vi "RTS Write Test Sequence.vi"(6 "Station Number":u16=1 min=1 max=8 step=1, 8 "Error In":errorcluster, 10 "Station Settings.Chamber Test Pattern":T1, 11 "Current Config File":T2 {"Chamber 1-1"."Start Time" format="%<%X\n%x>T"; "Chamber 1-1"."End Time" format="%<%X\n%x>T"; "Chamber 1-2"."Start Time" format="%<%X\n%x>T"; "Chamber 1-2"."End Time" format="%<%X\n%x>T"; "Chamber 1-3"."Start Time" format="%<%X\n%x>T"; "Chamber 1-3"."End Time" format="%<%X\n%x>T"}) -> (0 "Error Out":errorcluster)   [LabVIEW 2020]
uses:
  Type Definitions/RTS Door Op Data.ctl
  Type Definitions/RTS Door Ops Client.ctl
  Type Definitions/RTS Door Opening Schedule.ctl
  Type Definitions/RTS Door Ops Sequence.ctl
  Type Definitions/RTS Standard Door Opening Test.ctl
  Type Definitions/RTS Test Pattern.ctl
  <vilib>/Utility/config.llb/NI_LVConfig.lvlib
panel:
  # "Chamber Conditions:"
  # "Chamber Conditions:"
  # "Chamber Conditions:"
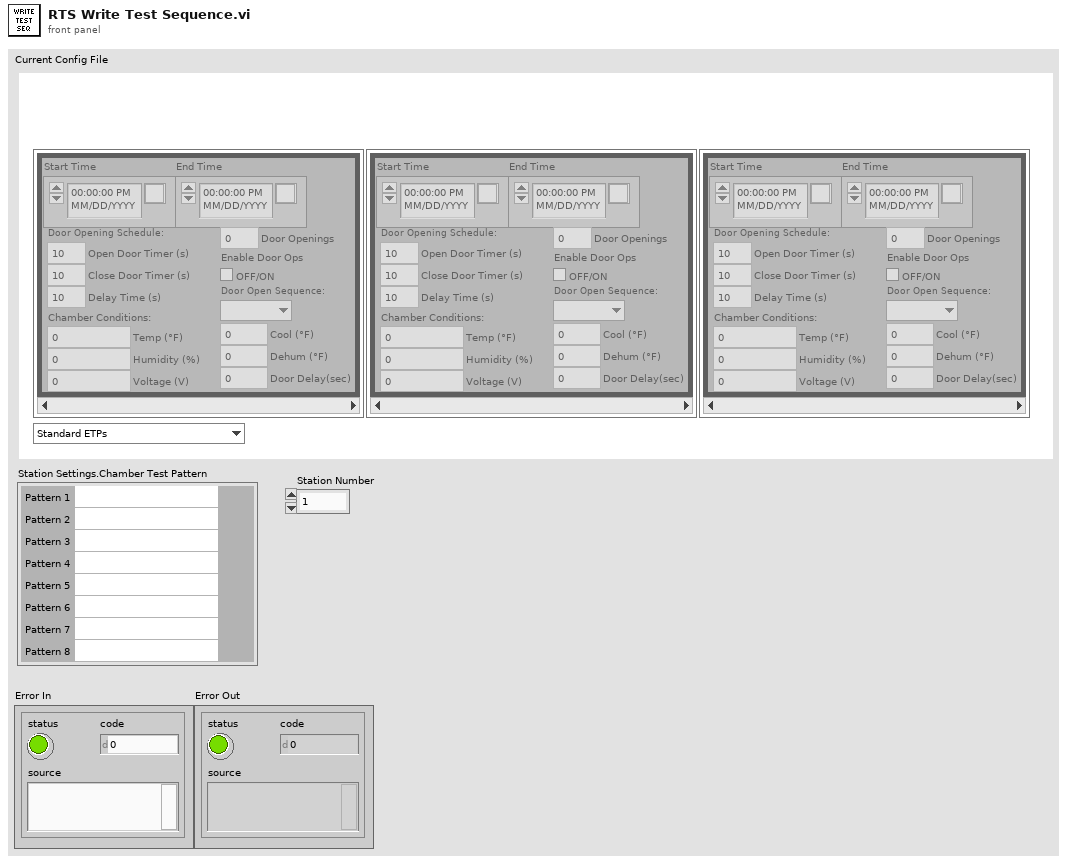
[diagram p1: front panel]
types:
  T1 = typedef "RTS Test Pattern.ctl" = cluster{" Pattern 1":path, "Pattern 2":path, "Pattern 3":path, "Pattern 4":path, "Pattern 5":path, "Pattern 6":path, "Pattern 7":path, "Pattern 8":path}
  T2 = typedef "RTS Door Op Data.ctl" = cluster{"Chamber 1-3":T3[], "Chamber 1-2":T3[], "Chamber 1-1":T3[], "Standard Tests 1-1":T6}
  T3 = typedef "RTS Door Ops Client.ctl" = cluster{"End Time":timestamp, "Start Time":timestamp, "Door Opening Schedule:":T4, "Enable Door Ops":bool, "Door Openings":u32, "Temp (°F)":dbl, "Humidity (%)":dbl, "Voltage (V)":dbl, "Door Open Sequence:":T5, "Door Delay(sec)":dbl, "Dehum (°F)":dbl, "Cool (°F)":dbl}
  T4 = typedef "RTS Door Opening Schedule.ctl" = cluster{"Open Door Timer (s)":dbl, "Delay Time (s)":dbl, "Close Door Timer (s)":dbl}
  T5 = typedef "RTS Door Ops Sequence.ctl" = enum16{"", "1st", "2nd", "3rd"}
  T6 = typedef "RTS Standard Door Opening Test.ctl" = enum16{"Standard ETPs", "511-B113 EHUT", "511-B110 HUT", "512-C410 SLAT", "511-B111 Internal Moisture", "511-C401 Moisture Accumulation", "511-B100 No Door Opening (NDO)", "511-B304 ISO Energy Consumption", "Custom Test", "Cancel Test"}
  T7 = typedef "NI_LVConfig.lvlib/Config Data RefNum.ctl" = refnum<k1>
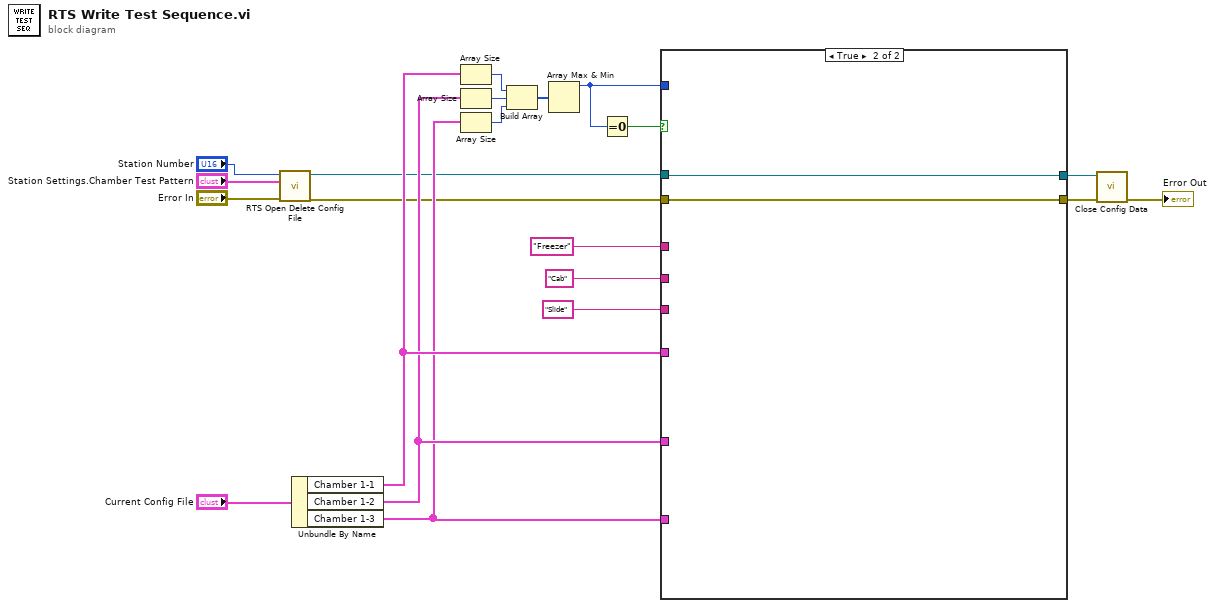
[diagram p0: block diagram]
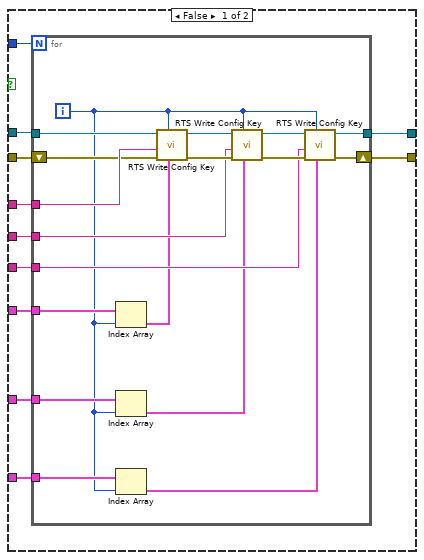
[diagram p2: hidden frame]
diagram:
  n1 = call "RTS Open Delete Config File.vi"("error in (no error)"="Error In", "Station Settings.Chamber Test Pattern"="Station Settings.Chamber Test Pattern", "Station Number"="Station Number") -> ("Error Out"=w5:errorcluster, "Refnum out"=w4:T7)  [unwired: 7 in]
  n2 = Unbundle By Name("Current Config File") -> ("Chamber 1-1"=w8:T3[], "Chamber 1-2"=w7:T3[], "Chamber 1-3"=w6:T3[])
  n3 = Array Size(array=w8) -> (size(s)=w10:i32)
  n4 = Array Size(array=w7) -> (size(s)=w11:i32)
  n5 = Array Size(array=w6) -> (size(s)=w9:i32)
  n6 = Build Array(w10, w11, w9) -> (w12:i32[])
  n7 = Array Max & Min(array=w12) -> (max value=w2:i32)  [unwired: 3 out]
  n8 = Equal To 0?(x=w2) -> (x = 0?=w1:bool)
  n9 = case shown="True" w1 {
    tunnel: [w32 w52] -> w20
    tunnel: [w31 w51] -> w19
    tunnel: "Freezer" -> [w30 _]
    tunnel: "Cab" -> [w29 _]
    tunnel: "Slide" -> [w28 _]
    tunnel: w8 -> [w27 _]
    tunnel: w7 -> [w26 _]
    tunnel: w6 -> [w25 _]
    tunnel: w5 -> [w24 w52]
    tunnel: w4 -> [w23 w51]
    tunnel: w2 -> [w22 _]
    frame False {
      n10 = for {
        N: w22 -> [_]
        tunnel: w27 -> [w39]
        shift-right: [w45] -> w32
        shift-left: w24 -> [w48]
        tunnel: [w42] -> w31
        tunnel: w23 -> [w49]
        tunnel: w30 -> [w50]
        tunnel: w29 -> [w41]
        tunnel: w28 -> [w40]
        tunnel: w26 -> [w37]
        tunnel: w25 -> [w35]
        i -> [w33]
        n11 = Index Array(array=w39, index=w33) -> (element=w38:T3)
        n12 = Index Array(array=w37, index=w33) -> (element=w36:T3)
        n13 = Index Array(array=w35, index=w33) -> (element=w34:T3)
        n14 = call "RTS Write Config Key.vi"("Chamber 1-1"=w38, "Loop Index"=w33, "error in (no error)"=w48, "Relay Name (Freezer, Cab,Slide)"=w50, "Refnum in"=w49) -> ("error out"=w47:errorcluster, "Refnum out"=w43:T7)  [unwired: 5 in]
        n15 = call "RTS Write Config Key.vi"("Chamber 1-1"=w36, "Loop Index"=w33, "error in (no error)"=w47, "Relay Name (Freezer, Cab,Slide)"=w41, "Refnum in"=w43) -> ("error out"=w46:errorcluster, "Refnum out"=w44:T7)  [unwired: 5 in]
        n16 = call "RTS Write Config Key.vi"("Chamber 1-1"=w34, "Loop Index"=w33, "error in (no error)"=w46, "Relay Name (Freezer, Cab,Slide)"=w40, "Refnum in"=w44) -> ("error out"=w45:errorcluster, "Refnum out"=w42:T7)  [unwired: 5 in]
      }
    }
    frame True {
    }
  }
  n17 = call <vilib>:"Close Config Data.vi"("error in (no error)"=w20, "refnum"=w19) -> ("error out"=→"Error Out":errorcluster)  [unwired: 1 in, 8 out]
